vi "loadModel.vi"(8 "Error In":errorcluster, 11 "UI Elements Cluster":T1) -> (0 "Error Out":errorcluster)   [LabVIEW 2018]
uses:
  UI Module/src/controls/mainAppElementsCluster.ctl
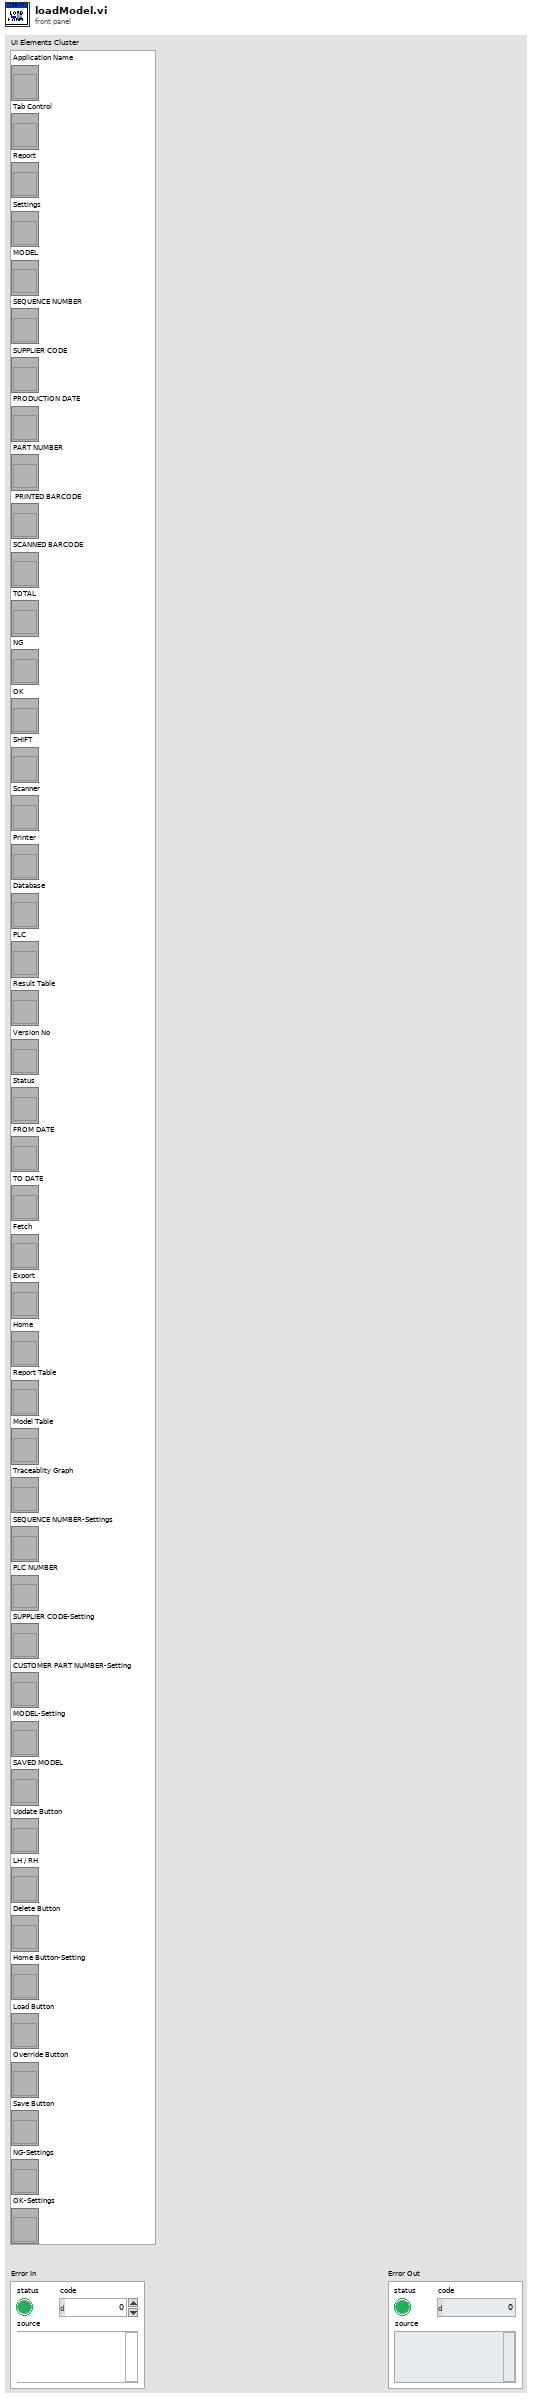
[diagram p1: front panel]
types:
  T1 = typedef "mainAppElementsCluster.ctl" = cluster{"Application Name":refnum<vi>, "Tab Control":refnum<vi>, "Status":refnum<vi>, "Version No":refnum<vi>, "Result Table":refnum<vi>, "PLC":refnum<vi>, "Database":refnum<vi>, "Printer":refnum<vi>, "Scanner":refnum<vi>, "SHIFT":refnum<vi>, "OK":refnum<vi>, "NG":refnum<vi>, "TOTAL":refnum<vi>, "SCANNED BARCODE":refnum<vi>, " PRINTED BARCODE":refnum<vi>, "PART NUMBER":refnum<vi>, "PRODUCTION DATE":refnum<vi>, "SUPPLIER CODE":refnum<vi>, "SEQUENCE NUMBER":refnum<vi>, "MODEL":refnum<vi>, "Settings":refnum<vi>, "Report":refnum<vi>, "Report Table":refnum<vi>, "Home":refnum<vi>, "Export":refnum<vi>, "Fetch":refnum<vi>, "TO DATE":refnum<vi>, "FROM DATE":refnum<vi>, "Model Table":refnum<vi>, "Traceablity Graph":refnum<vi>, "Override Button":refnum<vi>, "Load Button":refnum<vi>, "Home Button-Setting":refnum<vi>, "Delete Button":refnum<vi>, "Update Button":refnum<vi>, "Save Button":refnum<vi>, "SEQUENCE NUMBER-Settings":refnum<vi>, "PLC NUMBER":refnum<vi>, "LH / RH":refnum<vi>, "SUPPLIER CODE-Setting":refnum<vi>, "CUSTOMER PART NUMBER-Setting":refnum<vi>, "MODEL-Setting":refnum<vi>, "SAVED MODEL":refnum<vi>, "NG-Settings":refnum<vi>, "OK-Settings":refnum<vi>}
  T2 = cluster{"[0]":string, "[1]":string, "[2]":string, "[3]":string, "[4]":string, "[5]":string, "[6]":string, "[7]":string, "[8]":string}
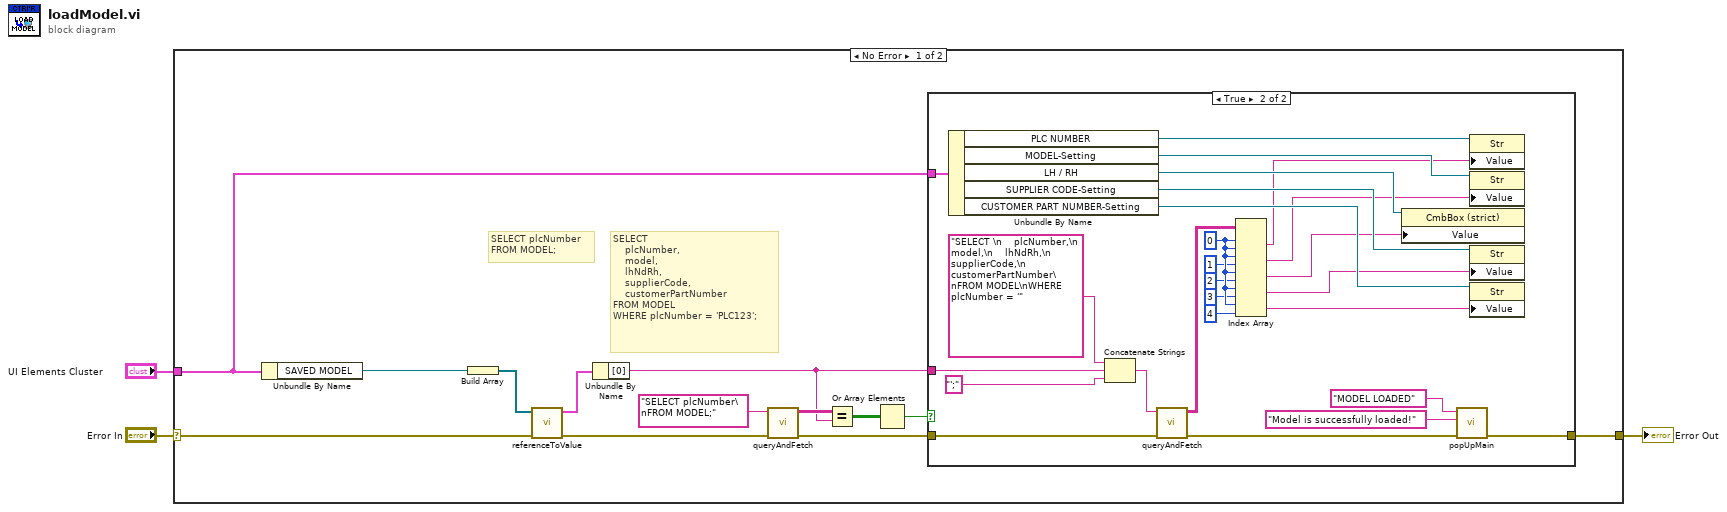
[diagram p0: block diagram]
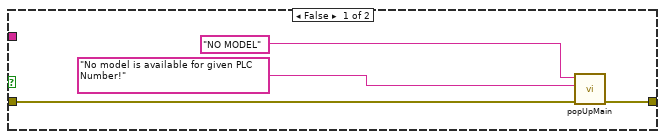
[diagram p2: hidden frame]
diagram:
  n1 = case shown="No Error" "Error In" {
    selector: "Error In" -> [w14 w47]
    tunnel: [w8 w47] -> w2
    tunnel: "UI Elements Cluster" -> [w5 _]
    frame No Error {
      # "SELECT \n    plcNumber,\n    model,\n    lhNdRh,\n    supplierCode,\n    customerPartNumber\nFROM MODEL\nWHERE plcNumber = 'PLC123';"
      # "SELECT plcNumber\nFROM MODEL;"
      n2 = Unbundle By Name(w5) -> ("SAVED MODEL"=w16:refnum<vi>)
      n3 = Build Array(w16) -> (w6:refnum<vi>[])
      n4 = call "referenceToValue.vi"("Error In"=w14, "Reference Array"=w6) -> ("Error Out"=w13:errorcluster, "Value Out Cluster"=w15:T2)  [unwired: 8 in]
      n5 = Unbundle By Name(w15) -> ("[0]"=w7:string)
      n6 = call "queryAndFetch.vi"("Error In"=w13, "Query"="SELECT plcNumber\nFROM MODEL;") -> ("Error Out"=w9:errorcluster, "Result Table"=w11:string[][])  [unwired: 8 in]
      n7 = Equal?(x=w11, y=w7) -> (x = y?=w10:bool[][])
      n8 = Or Array Elements(Boolean array=w10) -> (logical OR=w4:bool)
      n9 = case shown="True" w4 {
        tunnel: w9 -> [w20 w46]
        tunnel: [w19 w21] -> w8
        tunnel: w7 -> [_ w43]
        tunnel: w5 -> [_ w40]
        frame False {
          n10 = call "popUpMain.vi"("Error In"=w20, "Message Description"="No model is available for given PLC Number!" ("Error Info"), "Message Titlt"="NO MODEL" ("Error Name")) -> ("Error Out"=w19:errorcluster)  [unwired: 7 in, 1 out]
        }
        frame True {
          w34 = 0 ("index (row)")
          n11 = Unbundle By Name(w40) -> ("PLC NUMBER"=w39:refnum<vi>, "MODEL-Setting"=w38:refnum<vi>, "LH / RH"=w37:refnum<vi>, "SUPPLIER CODE-Setting"=w36:refnum<vi>, "CUSTOMER PART NUMBER-Setting"=w35:refnum<vi>)
          n12 = Concatenate Strings("SELECT \n    plcNumber,\n    model,\n    lhNdRh,\n    supplierCode,\n    customerPartNumber\nFROM MODEL\nWHERE plcNumber = '", w43, "';" ("string")) -> (w45:string)
          n13 = call "queryAndFetch.vi"("Error In"=w46, "Query"=w45) -> ("Error Out"=w22:errorcluster, "Result Table"=w41:string[][])  [unwired: 8 in]
          n14 = Index Array(array=w41, index (row) #1=w34, index (col) #1=w34, index (row) #2=w34, index (col) #2=1 ("disabled index (col)"), index (row) #3=w34, index (col) #3=2 ("disabled index (col)"), index (row) #4=w34, index (col) #4=3 ("disabled index (col)"), index (row) #5=w34, index (col) #5=4 ("disabled index (col)")) -> (element #1=w29:string, element #2=w28:string, element #3=w27:string, element #4=w26:string, element #5=w25:string)
          n15 = property class="CmbBox (strict)"(reference=w37, "Value"=w27) -> ()  [unwired: 1 in, 2 out]
          n16 = call "popUpMain.vi"("Error In"=w22, "Message Description"="Model is successfully loaded!" ("Error Info"), "Message Titlt"="MODEL LOADED" ("Error Name")) -> ("Error Out"=w21:errorcluster)  [unwired: 7 in, 1 out]
          n17 = property class="Str"(reference=w39, "Value"=w29) -> ()  [unwired: 1 in, 2 out]
          n18 = property class="Str"(reference=w38, "Value"=w28) -> ()  [unwired: 1 in, 2 out]
          n19 = property class="Str"(reference=w36, "Value"=w26) -> ()  [unwired: 1 in, 2 out]
          n20 = property class="Str"(reference=w35, "Value"=w25) -> ()  [unwired: 1 in, 2 out]
        }
      }
    }
    frame Error {
    }
  }
  "Error Out" <- w2
